vi "FIR Windowed Filter (obs).vi"(0 "sampling freq: fs":dbl=1.0 format="%0.2f", 1 "X":dbl[](array[numeric]), 2 "filter type":T1(ring), 7 "low cutoff freq: fl":dbl=0.125 format="%0.2f", 11 "high cutoff freq: fh":dbl=0.45 format="%0.2f", 12 "taps":i32=25 min=1, 14 "window":i32(ring) items=["None", "Hanning", "Hamming", "Triangular", "Blackman", "Exact Blackman", "Blackman-Harris", "Kaiser-Bessel", "Flat Top"]) -> (4 "Filtered X":dbl[](array[numeric]), 10 "error":i32)   [LabVIEW 2020, in "NI_AALBase.lvlib"]
doc: "Filters the input data sequence, <B>X</B>, using the set of windowed FIR filter coefficients specified by the <B>sampling freq: fs</B>, <B>low cutoff freq: fl</B>, <B>high cutoff freq: fh</B>, and number of <B>taps</B>."
uses:
  NI_AALBase.lvlib
  NI_AALPro.lvlib
panel:
  # "This VI is obsolete !!!\nYou should replace this VI in your diagram with the FIR Windowed Filter VI.  \n\nNOTE: If you have wired to the window input of this obsolete VI, \n           please be aware that the new FIR Window Filter VI has a different\n           window input."
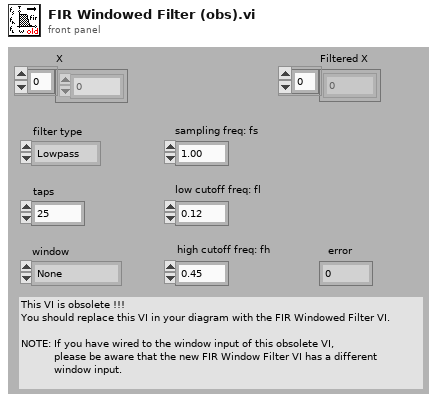
[diagram p1: front panel]
types:
  T1 = enum32{"Lowpass", "Highpass", "Bandpass", "Bandstop"}
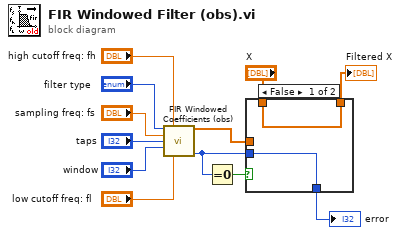
[diagram p0: block diagram]
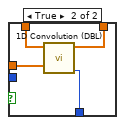
[diagram p2: hidden frame]
diagram:
  n1 = call "FIR Windowed Coefficients (obs).vi"("filter type"="filter type", "high cutoff freq: fh"="high cutoff freq: fh", "sampling freq: fs"="sampling freq: fs", "taps"="taps", "window"="window", "low cutoff freq: fl"="low cutoff freq: fl") -> ("FIR Windowed Coefficients"=w8:dbl[], "error"=w1:i32)  [unwired: 8 in]
  n2 = Equal To 0?(x=w1) -> (x = 0?=w2:bool)
  n3 = case shown="False" w2 {
    tunnel: [w14 w16] -> w11
    tunnel: w1 -> [w14 _]
    tunnel: "X" -> [w13 w18]
    tunnel: [w13 w17] -> w9
    tunnel: w8 -> [_ w15]
    frame False {
    }
    frame True {
      n4 = call "1D Convolution (DBL).vi"("Y"=w15, "X"=w18) -> ("error"=w16:i32, "X * Y"=w17:dbl[])  [unwired: 8 in]
    }
  }
  "Filtered X" <- w9
  "error" <- w11
